vi "Database-SQLiteCloseAllCallers.vi"(8 "error in (no error)":errorcluster, 11 "Database-Actor in":refnum<class "Database-Actor.lvclass">) -> (0 "error out":errorcluster, 3 "Database-Actor out":refnum<class "Database-Actor.lvclass">)   [LabVIEW 2013]
uses:
  ftw-dataflow/Core/utils/CodeGen/SQLite-Fetch/FTW-SQLite-Fetch.xnode
  ftw-dataflow/Actor/src/Connector/FTW-ActorConnector.lvclass
  ftw-dataflow/Core/src/Database/FTW-SQLite-PrepareStatement.vi
  ftw-dataflow/Core/src/Database/FTW-SQLite-Connector.lvclass
  ftw-dataflow/Core/src/Database/FTW-SQLite-LibraryReturnValue.vi
  ftw-dataflow/Core/src/Error/FTW-ERR-StatusOK.vi
  ftw-dataflow/Core/src/Error/FTW-ERR-ThrowImpossibleError.vi
  ftw-dataflow/Core/src/Database/FTW-SQLite-LibraryFilepath.vi
  ftw-dataflow/Core/src/Time/FTW-Time-Uptime.vi
  Database-Actor.lvclass
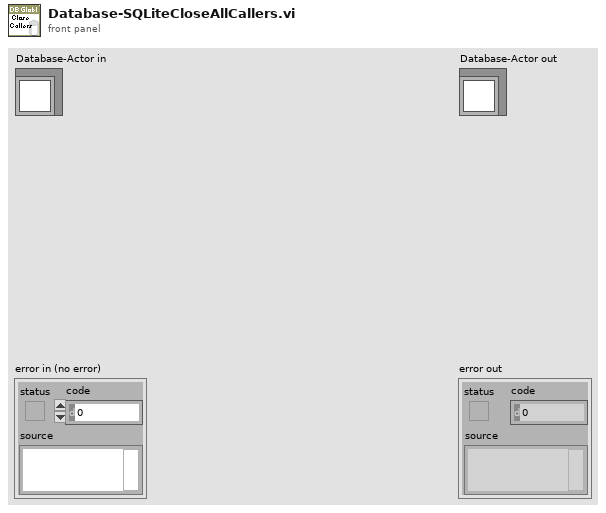
[diagram p1: front panel]
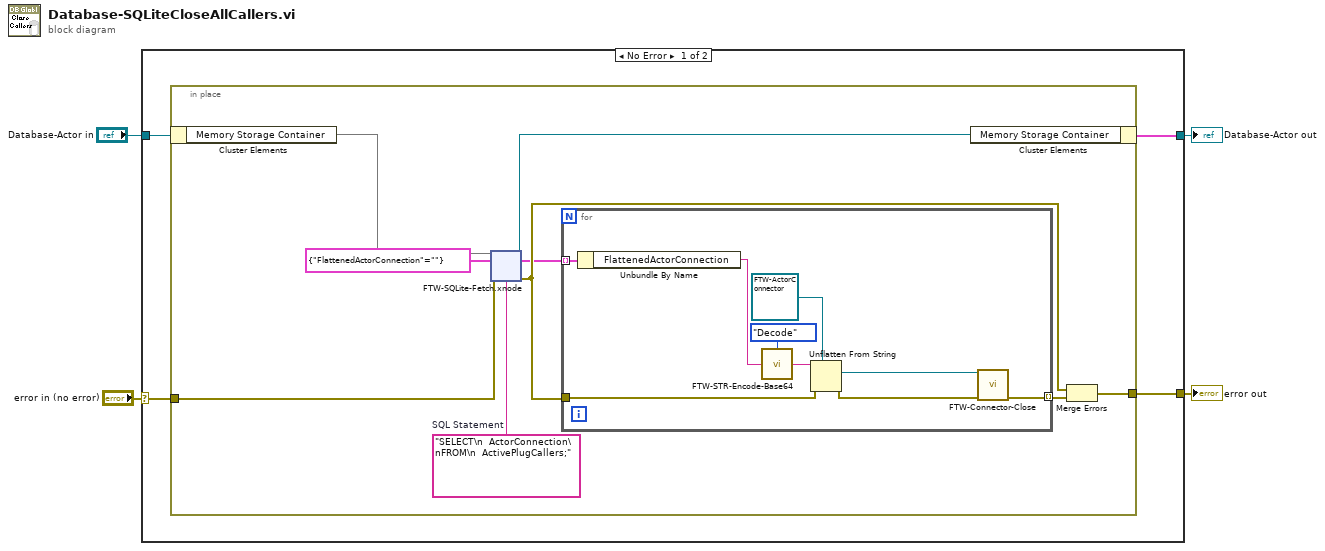
[diagram p0: block diagram]
diagram:
  n1 = case shown="No Error" "error in (no error)" {
    selector: "error in (no error)" -> [w8 w140]
    tunnel: [w7 w140] -> w3
    tunnel: [w5 w139] -> w1
    tunnel: "Database-Actor in" -> [w6 w139]
    frame No Error {
      n2 = in-place {
        in-place-border: w8 -> [w10]
        in-place-border: [w9] -> w7
        w14 = "SELECT\n  ActorConnection\nFROM\n  ActivePlugCallers;"  # SQL Statement
        n3 = in-place-cluster #1(w6) -> ("Memory Storage Container"=w12)
        n4 = xnode "FTW-SQLite-Fetch.xnode"("SQLite Connector"=w12, "SQL Script"=w14, "Row Datatype"=cluster{"FlattenedActorConnection":string} {"FlattenedActorConnection"=""}, "error in"=w10) -> ("SQLite Connector out"=w13:refnum<class "FTW-SQLite-Connector.lvclass">, "Result Set"=w15:cluster{"FlattenedActorConnection":string}[], "error out"=w17:errorcluster)  [unwired: 2 out]
        n5 = for {
          tunnel: w15 -> [w26] mode=indexing
          tunnel: w17 -> [w22]
          tunnel: [w20] -> w16 mode=indexing
          n6 = Unbundle By Name(w26) -> ("FlattenedActorConnection"=w25:string)
          n7 = call "FTW-STR-Encode-Base64.vi"("Input"=w25, "Direction"=enum16{"Encode", "Decode"}."Decode") -> ("Output"=w23:string)
          n8 = Unflatten From String(type=refnum<class "FTW-ActorConnector.lvclass"> refnum ("Featherweight Actor:FTW Actor Connector"), binary string=w23, error in (no error)=w22) -> (value=w19:refnum<class "FTW-ActorConnector.lvclass">, error out=w18:errorcluster)  [unwired: 2 in, 1 out]
          n9 = call-dynamic "FTW-Connector-Close.vi"("FTW Actor Connector"=w19, "error in"=w18) -> ("error out"=w20:errorcluster)  [unwired: 13 in]
        }
        n10 = in-place-cluster #1("Memory Storage Container"=w13) -> (w5:cluster{})
        n11 = Merge Errors(w17, w16) -> (w9:errorcluster)
      }
    }
    frame Error {
    }
  }
  "error out" <- w3
  "Database-Actor out" <- w1
